vi "Main_rownolegle.vi"() -> ()   [LabVIEW 2013]
doc: "Use this template to build a producer/consumer design pattern. Use this template when you need to execute a process, such as data analysis, when a data source, such as a triggered acquisition, produces data at an uneven rate and you need to execute the process when the data becomes available."
panel:
  out "data (can be any type)":string
  in  "Case Constant\n(See Context Help)":bool
  in  "stop":bool
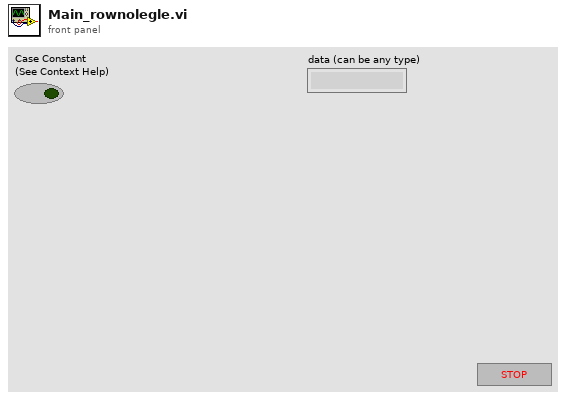
[diagram p1: front panel]
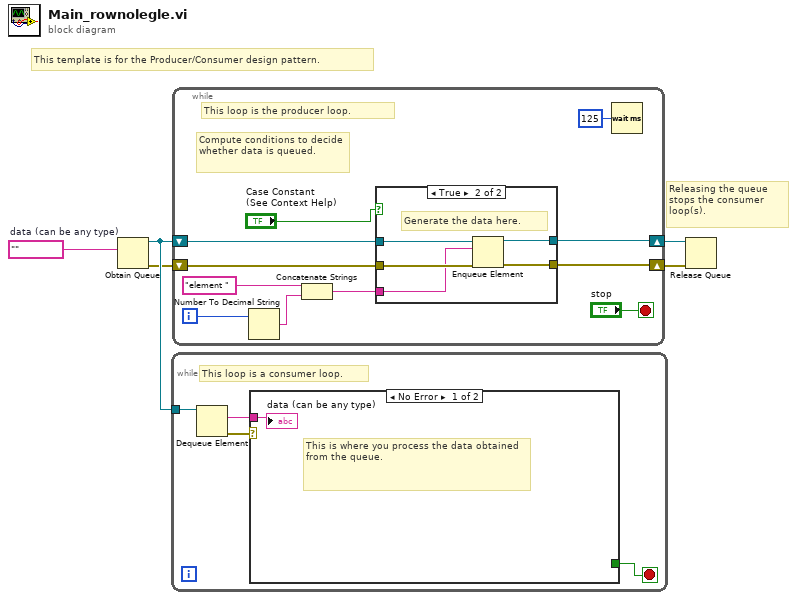
[diagram p0: block diagram]
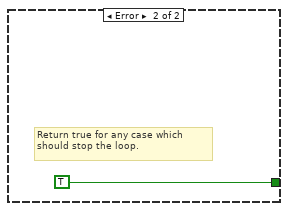
[diagram p2: hidden frame]
diagram:
  w1 = ""  # data (can be any type)
  # "Releasing the queue stops the consumer loop(s)."
  # "This template is for the Producer/Consumer design pattern."
  n1 = Obtain Queue(element data type=w1) -> (queue out=w5:refnum<queue>, error out=w4:errorcluster)  [unwired: 4 in, 1 out]
  n2 = while {
    tunnel: w5 -> [w9]
    stop <- w6 stop-if-true
    # "This loop is a consumer loop."
    n3 = Dequeue Element(queue=w9) -> (element=w7:string, error out=w8:errorcluster)  [unwired: 2 in, 2 out]
    n4 = case shown="No Error" w8 {
      tunnel: w7 -> [w10 _]
      tunnel: [_ TRUE] -> w6
      frame No Error {
        # "This is where you process the data obtained from the queue."
        "data (can be any type)" <- w10
      }
      frame Error {
        # "Return true for any case which should stop the loop."
      }
    }
  }
  n5 = while {
    shift-right: [w18] -> w2
    shift-left: w4 -> [w19]
    shift-right: [w20] -> w3
    shift-left: w5 -> [w21]
    i -> [w13]
    stop <- "stop" stop-if-true
    # "Compute conditions to decide whether data is queued."
    # "This loop is the producer loop."
    n6 = Number To Decimal String(number=w13) -> (decimal integer string=w12:string)  [unwired: 1 in]
    n7 = Concatenate Strings "Concatenate Strings"("element " ("element"), w12) -> (w14:string)
    n8 = case shown="True" "Case Constant\n(See Context Help)" {
      tunnel: w21 -> [w24 w29]
      tunnel: [w24 w28] -> w20
      tunnel: w19 -> [w23 w27]
      tunnel: [w23 w26] -> w18
      tunnel: w14 -> [_ w25]
      frame False {
      }
      frame True {
        # "Generate the data here."
        n9 = Enqueue Element(queue=w29, element=w25, error in (no error)=w27) -> (queue out=w28:refnum<queue>, error out=w26:errorcluster)  [unwired: 1 in, 1 out]
      }
    }
    n10 = Wait (ms)(milliseconds to wait=u32 125) -> ()  [unwired: 1 out]
  }
  n11 = Release Queue(queue=w3, error in (no error)=w2) -> ()  [unwired: 1 in, 3 out]
